vi "Create.vi"(5 "Is Less Than in":refnum<class "Is Less Than.lvclass">, 8 "error in (no error)":errorcluster, 11 "Expected":variant) -> (0 "error out":errorcluster, 3 "Is Less Than":refnum<class "Is Less Than.lvclass">)   [LabVIEW 2017, in "Transparent Assertions.lvlib" / "Is Less Than.lvclass"]
uses:
  Is Less Than.lvclass
  Is Less Than.lvclass/Is Less Than.ctl
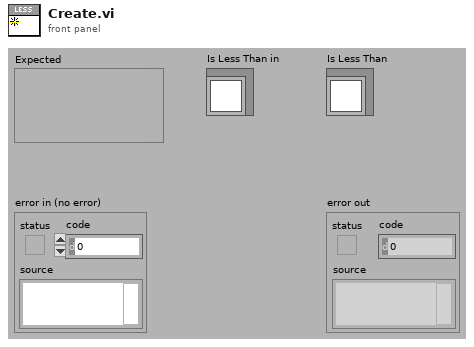
[diagram p1: front panel]
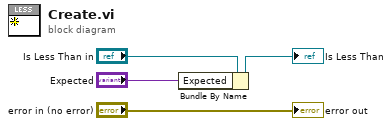
[diagram p0: block diagram]
diagram:
  n1 = Bundle By Name(cluster="Is Less Than in", "Expected"="Expected") -> (→"Is Less Than":refnum<class "Is Less Than.lvclass">)
  "error out" <- "error in (no error)"
